vi "Measure Cap_ERMod.vi"(8 "error in (no error)":errorcluster, 9 "VNAs Measurement Parameters":T2, 10 "Pins":string[](array[string])=["RF"], 11 "Semiconductor Module Context":T1) -> (0 "error out":errorcluster, 2 "Multisite Cap Data":dbl[][](array[numeric]), 3 "Semiconductor Module Context Out":T1)   [LabVIEW 2013]
uses:
  <vilib>/NI_TestStand_SemiconductorModule/NI_TestStand_Semiconductor_Module.lvlibp/PinMap/General/SemiconductorModuleContext.ctl
  VNAs Measurement Parameters.ctl
  Pin Map API/VNA Custom Instrument.lvlib
  <vilib>/NI_TestStand_SemiconductorModule/NI_TestStand_Semiconductor_Module.lvlibp
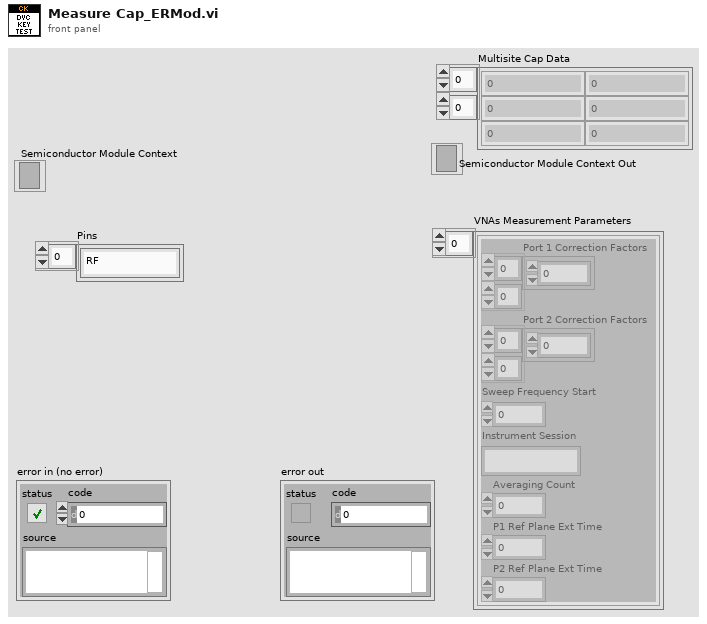
[diagram p1: front panel]
types:
  T1 = typedef "NI_TestStand_Semiconductor_Module.lvlibp/SemiconductorModuleContext.ctl" = refnum<k7>
  T2 = typedef "VNAs Measurement Parameters.ctl" = cluster{"Port 1 Correction Factors":cdb[][], "Port 2 Correction Factors":cdb[][], "Sweep Frequency Start":dbl, "Instrument Session":string, "Averaging Count":i32, "P1 Ref Plane Ext Time":dbl, "P2 Ref Plane Ext Time":dbl}[]
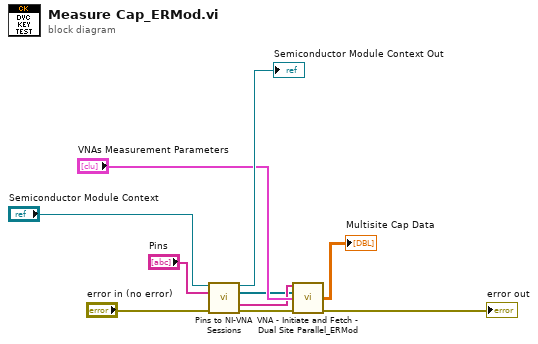
[diagram p0: block diagram]
diagram:
  n1 = call "Pins to NI-VNA Sessions.vi"("Semiconductor Module Context"="Semiconductor Module Context", "Pins"="Pins", "error in (no error)"="error in (no error)") -> ("Semiconductor Module Context Out"=→"Semiconductor Module Context Out":T1, "Instrument Sessions"=w1:refnum<k15>[], "Channel Lists"=w2:string[], "error out"=w6:errorcluster)  [unwired: 8 in, 1 out]
  n2 = call "VNA - Initiate and Fetch - Dual Site Parallel_ERMod.vi"("Channel Lists In"=w2, "Instrument Sessions In"=w1, "VNAs Measurement Parameters"="VNAs Measurement Parameters", "error in (no error)"=w6) -> ("Multisite Cap Data"=→"Multisite Cap Data":dbl[][], "error out"=→"error out":errorcluster)  [unwired: 6 in, 4 out]
